vi "SQL查询.vi"(7 "condition":string, 8 "error in (no error)":errorcluster, 9 "columns":string[](array[string]), 10 "table输入":string(combo), 11 "database":string(combo)) -> (0 "error out":errorcluster, 1 "拆分数据":bool, 2 "columns输出":string[](array[string]), 3 "data":string[][](table))   [LabVIEW 2016, in "数据传输系统-02.lvlib"]
uses:
  <vilib>/Utility/sysdir.llb/System Directory Type.ctl
  <vilib>/addons/database/Connection.llb/DB Tools Open Connec (String).vi
  <vilib>/addons/database/_DB Variant To Data/Database Variant To Data.xnode
  <vilib>/addons/database/NI_Database_API.lvlib
panel:
  out "error out 2":errorcluster
  out "结果字符串":string
  out "元素":string
  out "子数组":string[](array[string])
  # "时间 > #2021/01/15 08:00:00#and 时间 < #2021/04/15 08:00:00# order by 时间 asc"
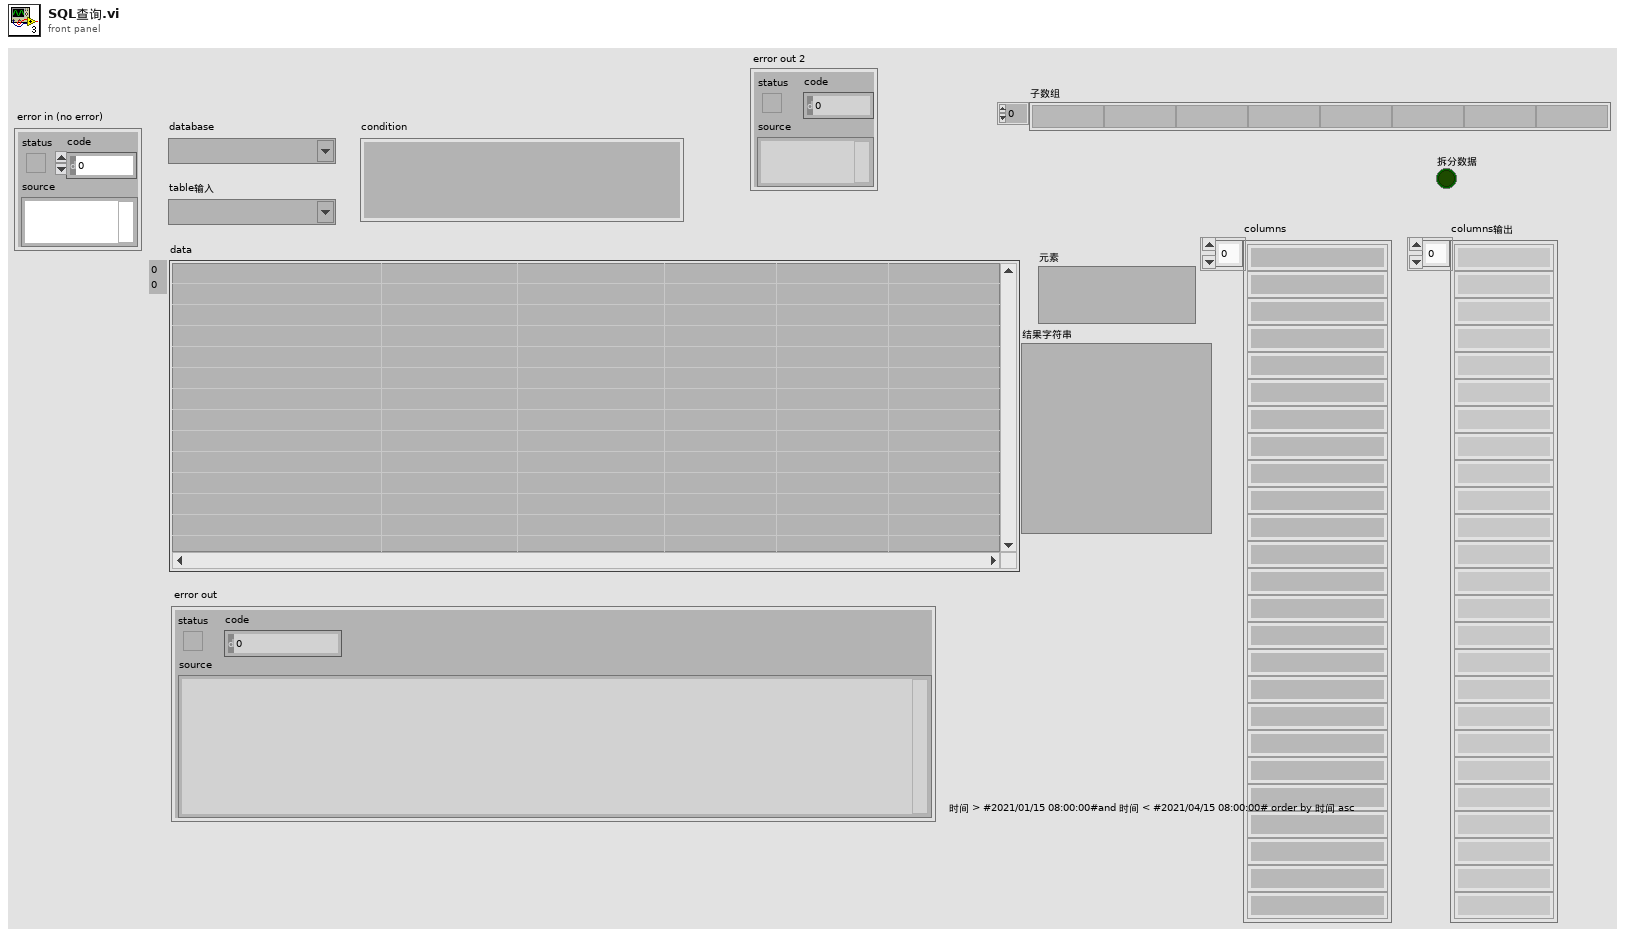
[diagram p1: front panel]
types:
  T1 = typedef "System Directory Type.ctl" = i32
  T2 = typedef "NI_Database_API.lvlib/Conn ObjectReference.ctl" = refnum<k1>
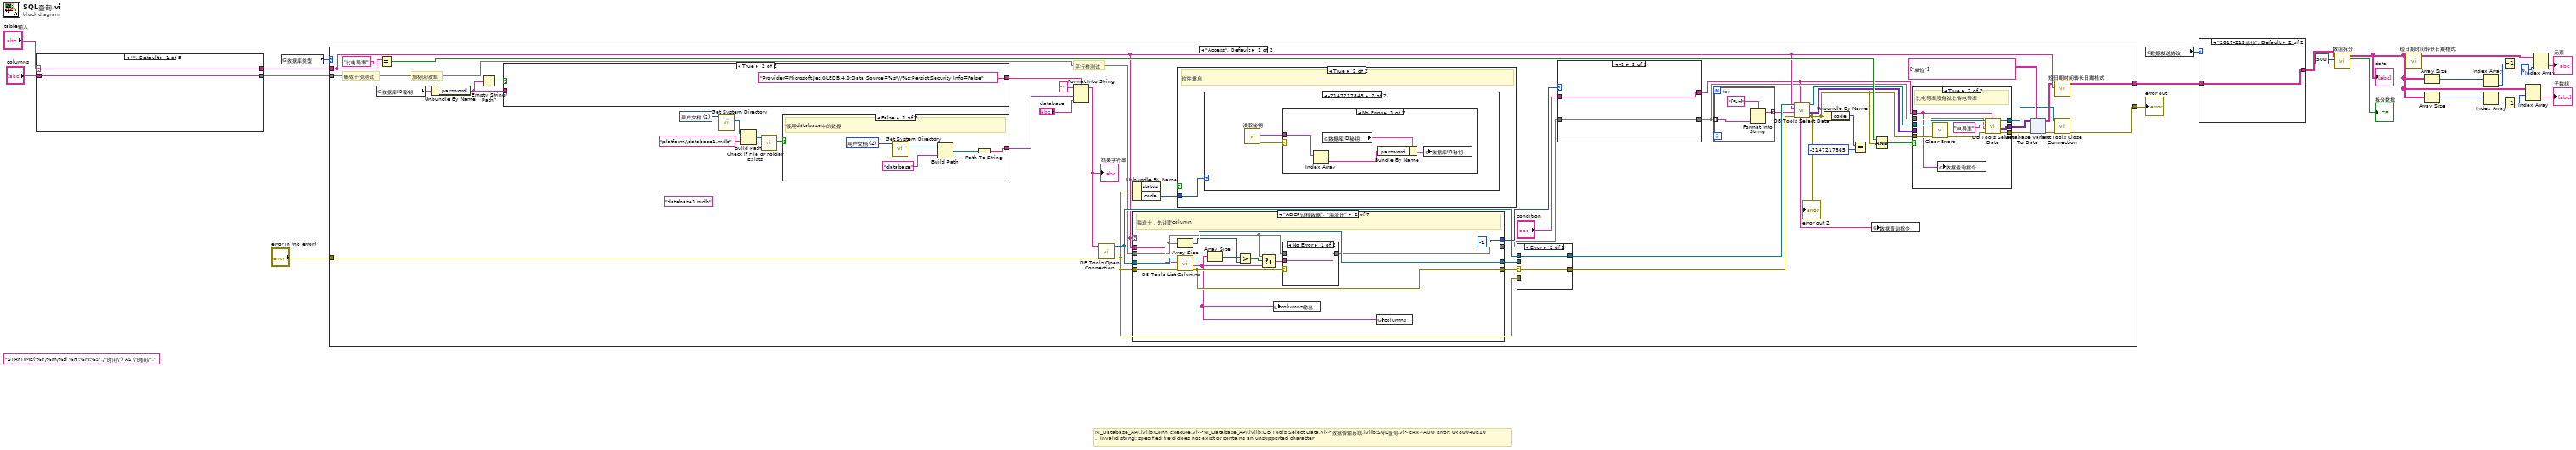
[diagram p0: block diagram]
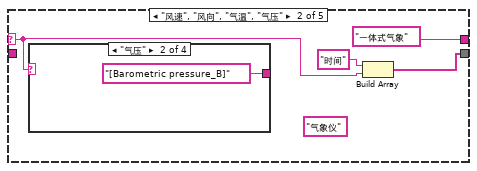
[diagram p2: hidden frame]
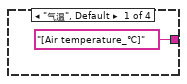
[diagram p3: hidden frame]
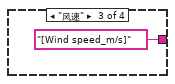
[diagram p4: hidden frame]
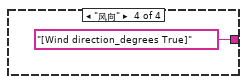
[diagram p5: hidden frame]
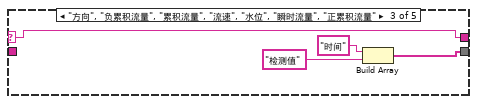
[diagram p6: hidden frame]
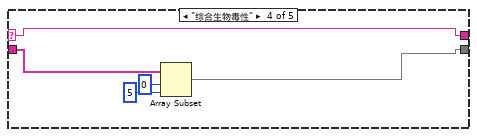
[diagram p7: hidden frame]
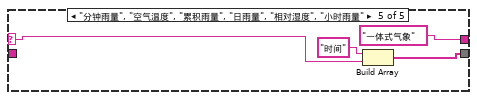
[diagram p8: hidden frame]
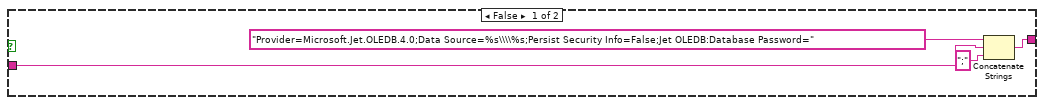
[diagram p9: hidden frame]
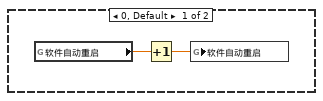
[diagram p11: hidden frame]
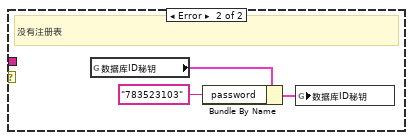
[diagram p12: hidden frame]
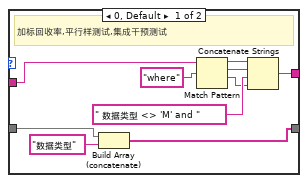
[diagram p13: hidden frame]
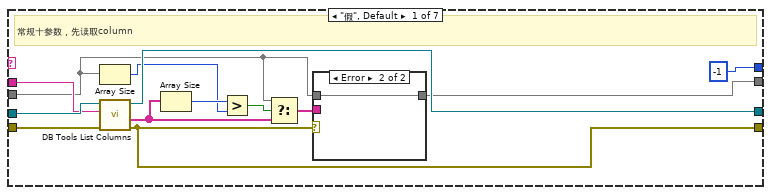
[diagram p15: hidden frame]
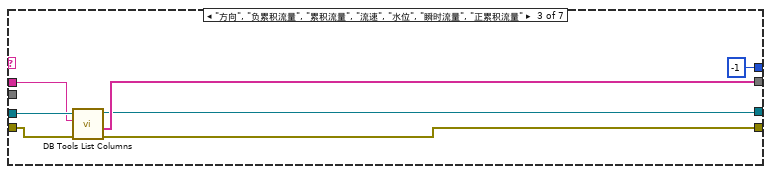
[diagram p18: hidden frame]
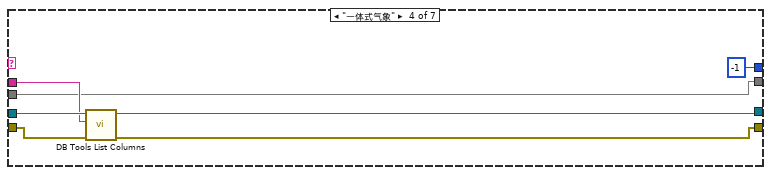
[diagram p19: hidden frame]
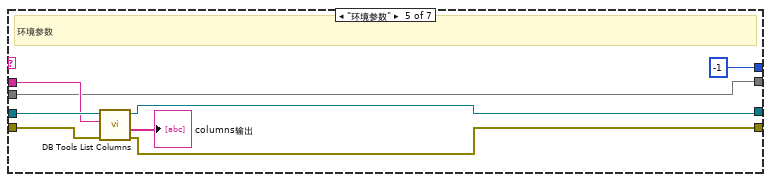
[diagram p20: hidden frame]
diagram:
  (unwired) "STRFTIME('%Y/%m/%d %H:%M:%S',\"时间\") AS \"时间\"," ("输入 1")
  # "NI_Database_API.lvlib:Conn Execute.vi->NI_Database_API.lvlib:DB Tools Select Data.vi->数据传输系统.lvlib:SQL查询.vi<ERR>ADO Error: 0x80040E10\n.  Invalid string: specified field does not exist or contains an unsupported character"
  n1 = case shown="\"\", Default" "table输入" {
    selector: "table输入" -> [w25 w27 w34 w42 w44]
    tunnel: [w25 "一体式气象" w34 w42 "一体式气象"] -> w4
    tunnel: "columns" -> [w24 _ _ w41 _]
    tunnel: [w24 w28 w36 w38 w45] -> w5
    frame "", Default {
    }
    frame "风速", "风向", "气温", "气压" {
      (unwired) "气象仪"
      n2 = case shown="\"气压\"" w27 {
        tunnel: ["[Air temperature_℃]" "[Barometric pressure_B]" "[Wind speed_m/s]" "[Wind direction_degrees True]"] -> _
        frame "气温", Default {
        }
        frame "气压" {
        }
        frame "风速" {
        }
        frame "风向" {
        }
      }
      n3 = Build Array("时间", w27) -> (w28:string[])
    }
    frame "方向", "负累积流量", "累积流量", "流速", "水位", "瞬时流量", "正累积流量" {
      n4 = Build Array("时间", "检测值") -> (w36:string[])
    }
    frame "综合生物毒性" {
      n5 = Array Subset(array=w41, index=0 ("索引"), length=5 ("长度")) -> (w38:string[])
    }
    frame "分钟雨量", "空气温度", "累积雨量", "日雨量", "相对湿度", "小时雨量" {
      n6 = Build Array("时间", w44) -> (w45:string[])
    }
  }
  n7 = global read "断电保存全局.vi" "数据库类型"() -> (w8:enum16{"Access", "SQLite"})
  n8 = case shown="\"Access\", Default" w8 {
    tunnel: [w90 w311] -> w23
    tunnel: [w66 w287] -> w11
    tunnel: "error in (no error)" -> [w61 w280]
    tunnel: w5 -> [w59 w283]
    tunnel: w4 -> [w58 w282]
    frame "Access", Default {
      (unwired) "database1.mdb" ("condition")
      w88 = T1 2 items=["用户目录"=0, "用户桌面"=1, "用户文档"=2, "用户应用程序数据"=3, "用户设置"=4, "用户临时目录"=5, "公共文档"=6, "公共应用程序数据"=7, "公共设置"=8, "公共缓存"=13, "系统核心库"=9, "系统安装库"=10, "应用程序文件"=11, "启动盘根目录"=12] ("system directory type")
      # "集成干预测试"
      # "平行样测试"
      # "加标回收率"
      n9 = global read "外部交互全局.vi" "数据库ID秘钥"() -> (w62:cluster{"userID":string, "password":string})
      n10 = Equal?(x=w58, y="比电导率") -> (x = y?=w84:bool)
      n11 = Unbundle By Name(w62) -> ("password"=w63:string)
      n12 = Empty String/Path?(string/path=w63) -> (empty?=w50:bool)
      n13 = case shown="True" w50 {
        tunnel: [w98 "Provider=Microsoft.Jet.OLEDB.4.0;Data Source=%s\\\\%s;Persist Security Info=False" ("格式字符串")] -> w64
        tunnel: w63 -> [w97 _]
        frame False {
          n14 = Concatenate Strings("Provider=Microsoft.Jet.OLEDB.4.0;Data Source=%s\\\\%s;Persist Security Info=False;Jet OLEDB:Database Password=" ("格式字符串"), w97, ";" ("字符串")) -> (w98:string)
        }
        frame True {
        }
      }
      n15 = call <vilib>:"Get System Directory.vi"("system directory type"=w88) -> ("system directory"=w89:path)  [unwired: 10 in]
      n16 = Build Path(base path=w89, name or relative path="platform\\database1.mdb" ("condition")) -> (appended path=w87:path)
      n17 = call <vilib>:"Check if File or Folder Exists.vi"("path"=w87) -> ("file or folder exists?"=w47:bool)  [unwired: 8 in, 2 out]
      n18 = case shown="False" w47 {
        tunnel: [w224 w229] -> w86
        frame False {
          w227 = T1 2 items=["用户目录"=0, "用户桌面"=1, "用户文档"=2, "用户应用程序数据"=3, "用户设置"=4, "用户临时目录"=5, "公共文档"=6, "公共应用程序数据"=7, "公共设置"=8, "公共缓存"=13, "系统核心库"=9, "系统安装库"=10, "应用程序文件"=11, "启动盘根目录"=12] ("system directory type")
          # "使用database中的数据"
          n19 = call <vilib>:"Get System Directory.vi"("system directory type"=w227) -> ("system directory"=w226:path)  [unwired: 10 in]
          n20 = Build Path(base path=w226, name or relative path="database" ("condition")) -> (appended path=w228:path)
          n21 = Path To String(path=w228) -> (string=w224:string)
        }
        frame True {
          w233 = T1 2 items=["用户目录"=0, "用户桌面"=1, "用户文档"=2, "用户应用程序数据"=3, "用户设置"=4, "用户临时目录"=5, "公共文档"=6, "公共应用程序数据"=7, "公共设置"=8, "公共缓存"=13, "系统核心库"=9, "系统安装库"=10, "应用程序文件"=11, "启动盘根目录"=12] ("system directory type")
          # "使用platform中的数据"
          n22 = call <vilib>:"Get System Directory.vi"("system directory type"=w233) -> ("system directory"=w232:path)  [unwired: 10 in]
          n23 = Build Path(base path=w232, name or relative path="platform" ("condition")) -> (appended path=w230:path)
          n24 = Path To String(path=w230) -> (string=w229:string)
        }
      }
      n25 = Format Into String(format string=w64, initial string="" ("初始字符串"), w86, "database") -> (resulting string=w54:string)  [unwired: 1 in, 1 out]
      "结果字符串" <- w54
      n26 = call-poly <vilib>:"DB Tools Open Connection.vi"("error in (no error)"=w61, "connection information"=w54) -> ("error out"=w51:errorcluster, "connection reference"=w70:T2)  [unwired: 6 in]
      n27 = Unbundle By Name(w51) -> ("status"=w65:bool, "code"=w57:i32)
      n28 = case shown="\"ADCP过程数据\", \"海流计\"" w58 {
        tunnel: w70 -> [w141 w156 w166 w173 w181 w189 w211]
        tunnel: w51 -> [w138 w153 w164 w172 w180 w188 w209]
        tunnel: [w139 w154 w161 w170 w179 w186 w208] -> w72
        tunnel: [w133 w149 w160 w169 w178 w187 w207] -> w73
        tunnel: w58 -> [w140 w155 w165 w171 w177 w190 w210]
        tunnel: [-1 ("index of element") -1 ("index of element") -1 ("index of element") -1 ("index of element") -1 ("index of element") -1 ("index of element") w204] -> w68
        tunnel: w59 -> [w130 w146 _ w167 w174 w185 w203]
        tunnel: [w131 w147 w163 w167 w174 w182 w203] -> w67
        frame "假", Default {
          # "常规十参数，先读取column"
          n29 = Array Size(array=w130) -> (size(s)=w135:i32)
          n30 = call <vilib>:"DB Tools List Columns.vi"("error in (no error)"=w138, "table"=w140, "connection reference"=w141) -> ("error out"=w133:errorcluster, "columns"=w134:string[], "connection reference out"=w139:T2)  [unwired: 1 in, 1 out]
          n31 = Array Size(array=w134) -> (size(s)=w136:i32)
          n32 = Greater?(x=w136, y=w135) -> (0:w137:bool)
          n33 = Select(t=w130, s=w137, f=w134) -> (s? t:f=w132:string[])
          n34 = case shown="Error" w133 {
            tunnel: w132 -> [w143 _]
            tunnel: [w143 w144] -> w131
            tunnel: w130 -> [_ w144]
            frame No Error {
            }
            frame Error {
            }
          }
        }
        frame "ADCP过程数据", "海流计" {
          # "海流计，先读取column"
          n35 = Array Size(array=w146) -> (size(s)=w150:i32)
          n36 = call <vilib>:"DB Tools List Columns.vi"("error in (no error)"=w153, "table"=w155, "connection reference"=w156) -> ("error out"=w149:errorcluster, "columns"=w145:string[], "connection reference out"=w154:T2)  [unwired: 1 in, 1 out]
          n37 = Array Size(array=w145) -> (size(s)=w151:i32)
          n38 = Greater?(x=w151, y=w150) -> (0:w152:bool)
          n39 = Select(t=w146, s=w152, f=w145) -> (s? t:f=w148:string[])
          n40 = local write "columns输出"(w145) -> ()
          n41 = case shown="No Error" w149 {
            tunnel: w148 -> [w158 _]
            tunnel: [w158 w159] -> w147
            tunnel: w146 -> [_ w159]
            frame No Error {
            }
            frame Error {
            }
          }
          n42 = global write "全局 所有参数.vi" "columns"(w145) -> ()
        }
        frame "方向", "负累积流量", "累积流量", "流速", "水位", "瞬时流量", "正累积流量" {
          n43 = call <vilib>:"DB Tools List Columns.vi"("error in (no error)"=w164, "table"=w165, "connection reference"=w166) -> ("error out"=w160:errorcluster, "columns"=w163:string[], "connection reference out"=w161:T2)  [unwired: 1 in, 1 out]
        }
        frame "一体式气象" {
          n44 = call <vilib>:"DB Tools List Columns.vi"("error in (no error)"=w172, "table"=w171, "connection reference"=w173) -> ("error out"=w169:errorcluster, "connection reference out"=w170:T2)  [unwired: 1 in, 2 out]
        }
        frame "环境参数" {
          # "环境参数"
          n45 = call <vilib>:"DB Tools List Columns.vi"("error in (no error)"=w180, "table"=w177, "connection reference"=w181) -> ("error out"=w178:errorcluster, "columns"=→"columns输出":string[], "connection reference out"=w179:T2)  [unwired: 1 in, 1 out]
        }
        frame "剖面数据" {
          # "环境参数"
          n46 = call <vilib>:"DB Tools List Columns.vi"("error in (no error)"=w188, "table"=w190, "connection reference"=w189) -> ("error out"=w187:errorcluster, "columns"=w184:string[], "connection reference out"=w186:T2)  [unwired: 1 in, 1 out]
          n47 = for {
            tunnel: w185 -> [w194] mode=indexing
            tunnel: w184 -> [w198]
            shift-right: [w192] -> w182
            shift-left: string[] [] -> [w195]
            n48 = Search 1D Array(1D array=w198, element=w194) -> (index of element=w197:i32)  [unwired: 1 in]
            n49 = Not Equal?(x=w197, y=-1) -> (x != y?=w193:bool)
            n50 = case shown="True" w193 {
              tunnel: w195 -> [w199 w202]
              tunnel: w194 -> [_ w201]
              tunnel: [w199 w200] -> w192
              frame False {
              }
              frame True {
                n51 = Build Array (concatenate)(w202, w201) -> (w200:string[])
              }
            }
          }
          n52 = local write "columns输出"(w182) -> ()
        }
        frame "集成干预测试", "加标回收率", "平行样测试" {
          n53 = call <vilib>:"DB Tools List Columns.vi"("error in (no error)"=w209, "table"=w210, "connection reference"=w211) -> ("error out"=w207:errorcluster, "columns"=w206:string[], "connection reference out"=w208:T2)  [unwired: 1 in, 1 out]
          n54 = Search 1D Array(1D array=w206, element="数据类型" ("元素")) -> (index of element=w204:i32)  [unwired: 1 in]
        }
      }
      n55 = case shown="True" w65 {
        tunnel: w57 -> [_ w102]
        frame False {
        }
        frame True {
          # "软件重启"
          n56 = case shown="-2147217843" w102 {
            frame 0, Default {
              n57 = global read "全局1.vi" "软件自动重启"() -> (w104:dbl)
              n58 = Increment(x=w104) -> (x+1=w103:dbl)
              n59 = global write "全局1.vi" "软件自动重启"(w103) -> ()
            }
            frame -2147217843 {
              n60 = call "读取秘钥.vi"() -> ("error out"=w105:errorcluster, "值"=w106:string[])  [unwired: 9 in, 1 out]
              n61 = case shown="No Error" w105 {
                tunnel: w106 -> [w110 _]
                frame No Error {
                  n62 = Index Array(array=w110) -> (element=w107:string)  [unwired: 1 in]
                  n63 = global read "外部交互全局.vi" "数据库ID秘钥"() -> (w108:cluster{"userID":string, "password":string})
                  n64 = Bundle By Name(cluster=w108, "password"=w107) -> (w109:cluster{"userID":string, "password":string})
                  n65 = global write "外部交互全局.vi" "数据库ID秘钥"(w109) -> ()
                }
                frame Error {
                  # "没有注册表"
                  n66 = global read "外部交互全局.vi" "数据库ID秘钥"() -> (w112:cluster{"userID":string, "password":string})
                  n67 = Bundle By Name(cluster=w112, "password"="783523103") -> (w113:cluster{"userID":string, "password":string})
                  n68 = global write "外部交互全局.vi" "数据库ID秘钥"(w113) -> ()
                }
              }
            }
          }
        }
      }
      n69 = case shown="Error" w73 {
        selector: w73 -> [_ w129]
        tunnel: w72 -> [w127 _]
        tunnel: [w127 w128] -> w71
        tunnel: w70 -> [_ w128]
        tunnel: [w126 w129] -> w69
        tunnel: w51 -> [w126 _]
        frame No Error {
        }
        frame Error {
        }
      }
      n70 = case "条件结构" shown="-1" w68 {
        tunnel: "condition" -> [w121 w124]
        tunnel: w67 -> [w123 w125]
        tunnel: [w115 w125] -> w56
        tunnel: [w114 w124] -> w49
        frame 0, Default {
          # "加标回收率,平行样测试,集成干预测试"
          n71 = Build Array (concatenate)(w123, "数据类型" ("元素")) -> (w115:string[])
          n72 = Match Pattern(string=w121, regular expression="where" ("正则表达式")) -> (before substring=w119:string, match substring=w118:string, after substring=w116:string)  [unwired: 1 in, 1 out]
          n73 = Concatenate Strings(w119, w118, " 数据类型 <> 'M' and " ("字符串"), w116) -> (w114:string)
        }
        frame -1 {
        }
      }
      n74 = for {
        tunnel: w56 -> [w96] mode=indexing
        tunnel: [w95] -> w55 mode=indexing
        n75 = Format Into String(format string="[%s]" ("格式字符串"), w96) -> (resulting string=w95:string)  [unwired: 2 in, 1 out]
      }
      n76 = call <vilib>:"DB Tools Select Data.vi"("condition"=w49, "error in (no error)"=w69, "columns"=w55, "table"=w58, "connection reference"=w71) -> ("error out"=w77:errorcluster, "data"=w79:variant[][], "connection reference out"=w82:T2)  [unwired: 1 in]
      "error out 2" <- w77
      n77 = Unbundle By Name(w77) -> ("code"=w76:i32)
      n78 = Equal?(x=w76, y=-2147217865 ("code")) -> (x = y?=w74:bool)
      n79 = global write "全局 水样时间.vi" "数据查询指令"(w49) -> ()
      n80 = Compound Arithmetic op=AND ("复合运算")(w84, w77, w74) -> (w83:bool)
      n81 = case shown="True" w83 {
        tunnel: w49 -> [_ w215]
        tunnel: w82 -> [w214 w223]
        tunnel: [w214 w218] -> w81
        tunnel: [w213 w219] -> w80
        tunnel: w79 -> [w213 _]
        tunnel: w77 -> [w212 w221]
        tunnel: [w212 w217] -> w78
        tunnel: w56 -> [_ w216]
        frame False {
        }
        frame True {
          # "比电导率没有就上传电导率"
          n82 = call <vilib>:"Clear Errors.vi"("error in (no error)"=w221) -> ("error out"=w220:errorcluster)  [unwired: 5 in, 1 out]
          n83 = global write "全局 水样时间.vi" "数据查询指令"(w215) -> ()
          n84 = call <vilib>:"DB Tools Select Data.vi"("condition"=w215, "error in (no error)"=w220, "columns"=w216, "table"="电导率", "connection reference"=w223) -> ("error out"=w217:errorcluster, "data"=w219:variant[][], "connection reference out"=w218:T2)  [unwired: 1 in]
        }
      }
      n85 = xnode "Database Variant To Data"("database variant"=w80, "error in (no error)"=w78, "type"=string[][] [["单位"]]) -> ("data"=w53:string[][], "error out"=w91:errorcluster)
      n86 = call "短日期时间转长日期格式.vi"("table输入"=w58, "data"=w53) -> ("输出数组"=w90:string[][])  [unwired: 9 in]
      n87 = call <vilib>:"DB Tools Close Connection.vi"("error in (no error)"=w91, "connection reference"=w81) -> ("error out"=w66:errorcluster)  [unwired: 5 in]
    }
    frame "SQLite" {
      w285 = "比电导率" ("y")
      (unwired) "order by STRFTIME('%Y/%m/%d %H:%M:%S',\"时间\")" ("替换字符串(\"\")")
      (unwired) "order by 时间" ("搜索字符串")
      w296 = TRUE ("替换全部？(F)")
      w313 = T1 2 items=["用户目录"=0, "用户桌面"=1, "用户文档"=2, "用户应用程序数据"=3, "用户设置"=4, "用户临时目录"=5, "公共文档"=6, "公共应用程序数据"=7, "公共设置"=8, "公共缓存"=13, "系统核心库"=9, "系统安装库"=10, "应用程序文件"=11, "启动盘根目录"=12] ("system directory type")
      n88 = local write "columns输出"(w283) -> ()
      n89 = local read "condition"() -> (w295:string)
      n90 = case shown="\"假\", Default" w282 {
        tunnel: w295 -> [w327 w333]
        tunnel: w283 -> [w326 w335]
        tunnel: [w326 w334] -> w306
        tunnel: [w327 w332] -> w294
        frame "假", Default {
        }
        frame "集成干预测试", "加标回收率", "平行样测试" {
          n91 = Build Array (concatenate)(w335, "数据类型" ("元素")) -> (w334:string[])
          n92 = call "数据库加密匹配 (子VI).vi"("输入参数"="N") -> ("Encoded String"=w330:string)  [unwired: 10 in]
          n93 = Match Pattern(string=w333, regular expression="where" ("正则表达式")) -> (before substring=w338:string, match substring=w337:string, after substring=w336:string)  [unwired: 1 in, 1 out]
          n94 = Format Into String(format string=" 数据类型 = '%s' and " ("字符串"), w330) -> (resulting string=w328:string)  [unwired: 2 in, 1 out]
          n95 = Concatenate Strings(w338, w337, w328, w336) -> (w332:string)
        }
      }
      n96 = local read "database"() -> (w298:string)
      n97 = Array Size(array=w306) -> (size(s)=w310:i32)
      n98 = call <vilib>:"Get System Directory.vi"("system directory type"=w313) -> ("system directory"=w312:path)  [unwired: 10 in]
      n99 = Search and Replace String(replace all?=w296, input string=w294, search string="/" ("搜索字符串"), replace string="-" ("替换字符串(\"\")")) -> (result string=w303:string)  [unwired: 4 in, 3 out]
      n100 = Equal To 0?(x=w310) -> (x = 0?=w309:bool)
      n101 = Build Path(base path=w312, name or relative path="Platform\\database1.db" ("condition")) -> (appended path=w314:path)
      n102 = case shown="False" w309 {
        tunnel: w306 -> [_ w343]
        tunnel: ["*" ("t") w342] -> w307
        frame True {
        }
        frame False {
          n103 = call <userlib>:"SQLite_Implode 1D.vi"("Values"=w343, "format string"="%s") -> ("imploded string"=w342:string)  [unwired: 7 in, 1 out]
        }
      }
      n104 = call <vilib>:"Check if File or Folder Exists.vi"("path"=w314) -> ("file or folder exists?"=w316:bool)  [unwired: 8 in, 2 out]
      n105 = Search and Replace String(replace all?=TRUE ("替换全部？(F)"), input string=w298, search string=".mdb" ("搜索字符串"), replace string=".db" ("替换字符串(\"\")")) -> (result string=w293:string)  [unwired: 4 in, 3 out]
      n106 = Search and Replace String(replace all?=w296, input string=w303, search string="#" ("搜索字符串"), replace string="'" ("替换字符串(\"\")")) -> (result string=w278:string)  [unwired: 4 in, 3 out]
      n107 = case shown="False" w316 {
        tunnel: [w346 w347] -> w281
        tunnel: w293 -> [w345 w348]
        frame False {
          # "使用database中的数据"
          n108 = call "database path.vi"("database"=w345) -> ("Path out"=w346:string)  [unwired: 9 in, 1 out]
        }
        frame True {
          # "使用platform中的数据"
          n109 = call "database platform path.vi"("database"=w348) -> ("Path out"=w347:string)  [unwired: 10 in]
        }
      }
      n110 = Format Into String(format string="SELECT %s %s FROM `%s` %s;" ("SQL Query"), "", w307, w282, w278) -> (resulting string=w288:string)  [unwired: 2 in, 1 out]
      n111 = call "Sqlite Query.vi"("DB Path"=w281, "SQL Query"=w288, "error in (no error)"=w280) -> ("Results"=w290:string[][], "DB Path Out"=w284:string, "error out"=w286:errorcluster)  [unwired: 10 in]
      n112 = Equal?(x=w282, y=w285) -> (x = y?=w292:bool)
      n113 = And(x=w286, y=w292) -> (x .and. y?=w291:bool)
      n114 = case shown="True" w291 {
        tunnel: w290 -> [w318 _]
        tunnel: [w318 w325] -> w289
        tunnel: w288 -> [_ w322]
        tunnel: w284 -> [_ w324]
        tunnel: [w317 w323] -> w287
        tunnel: w286 -> [w317 _]
        tunnel: w285 -> [_ w321]
        frame False {
        }
        frame True {
          n115 = Search and Replace String(input string=w322, search string=w321, replace string="电导率" ("Tables Name")) -> (result string=w319:string)  [unwired: 5 in, 3 out]
          n116 = call "Sqlite Query.vi"("DB Path"=w324, "SQL Query"=w319) -> ("Results"=w325:string[][], "error out"=w323:errorcluster)  [unwired: 11 in, 1 out]
        }
      }
      n117 = call "短日期时间转长日期格式.vi"("data"=w289) -> ("输出数组"=w311:string[][])  [unwired: 10 in]
    }
  }
  "error out" <- w11
  n118 = global read "断电保存全局.vi" "数据发送协议"() -> (w22:enum16{"2005-212协议", "2017-212协议"})
  n119 = case shown="\"2017-212协议\", Default" w22 {
    tunnel: w23 -> [w350 w357]
    tunnel: [w349 w357] -> w9
    frame "2005-212协议" {
      n120 = for {
        N: 1 -> [_]
        tunnel: string[][] [] ("data") -> [w356]
        tunnel: w350 -> [w355] mode=indexing
        tunnel: [w353] -> w349
        n121 = Insert Into Array(array=w356, index (row)=0 ("索引 (行)"), new element=w355) -> (w353:string[][])  [unwired: 1 in]
      }
    }
    frame "2017-212协议", Default {
    }
  }
  n122 = call "数组拆分.vi"("拆分大小"=500, "输入数据"=w9) -> ("拆分数据"=→"拆分数据":bool, "输出数组"=w1:string[][])  [unwired: 8 in]
  "data" <- w1
  n123 = call "短日期时间转长日期格式.vi"("data"=w1) -> ("输出数组"=w17:string[][])  [unwired: 10 in]
  n124 = Array Size(array=w1) -> (size(s)=w16:i32[])
  n125 = Array Size(array=w1) -> (size(s)=w21:i32[])
  n126 = Index Array(array=w16) -> (element=w15:i32)  [unwired: 1 in]
  n127 = Index Array(array=w21) -> (element=w19:i32)  [unwired: 1 in]
  n128 = Decrement(x=w15) -> (x-1=w14:i32)
  n129 = Decrement(x=w19) -> (x-1=w18:i32)
  n130 = Index Array(array=w1, index (row)=w18) -> (element=→"子数组":string[])  [unwired: 1 in]
  n131 = Index Array(array=w17, index (row)=w14, index (col)=0 ("禁用的索引 (列)")) -> (element=→"元素":string)
